vi "Komparator 4.0..vi"(10 "Q":u8, 11 "P":u8) -> (2 "P>Q":bool, 3 "P=Q":bool)   [LabVIEW 2020]
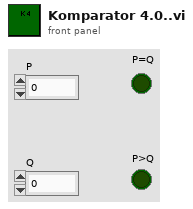
[diagram p1: front panel]
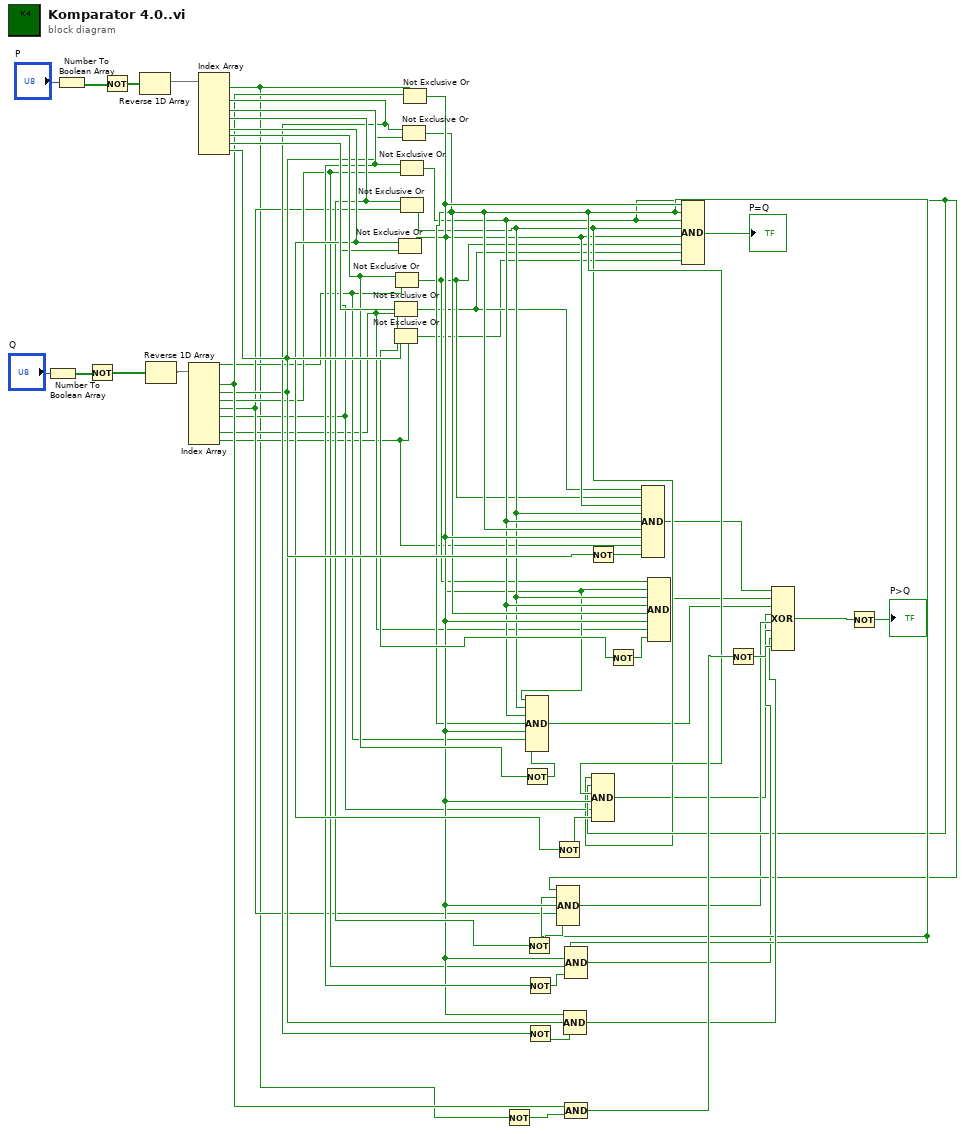
[diagram p0: block diagram]
diagram:
  n1 = Number To Boolean Array(number="Q") -> (Boolean array=w5:bool[])
  n2 = Number To Boolean Array(number="P") -> (Boolean array=w4:bool[])
  n3 = Not(x=w5) -> (.not. x?=w7:bool[])
  n4 = Not(x=w4) -> (.not. x?=w6:bool[])
  n5 = Reverse 1D Array(array=w6) -> (reversed array=w10:bool[])
  n6 = Reverse 1D Array(array=w7) -> (reversed array=w9:bool[])
  n7 = Index Array "Index Array"(array=w9) -> (element #1=w33:bool, element #2=w32:bool, element #3=w29:bool, element #4=w26:bool, element #5=w23:bool, element #6=w20:bool, element #7=w16:bool, element #8=w14:bool)  [unwired: 8 in]
  n8 = Index Array "Index Array"(array=w10) -> (element #1=w1:bool, element #2=w35:bool, element #3=w37:bool, element #4=w39:bool, element #5=w41:bool, element #6=w43:bool, element #7=w47:bool, element #8=w49:bool)  [unwired: 8 in]
  n9 = Not Exclusive Or(1:w16, 2:w47) -> (0:w13:bool)
  n10 = Not Exclusive Or(1:w14, 2:w49) -> (0:w11:bool)
  n11 = Not Exclusive Or(1:w20, 2:w43) -> (0:w15:bool)
  n12 = Not Exclusive Or(1:w23, 2:w41) -> (0:w19:bool)
  n13 = Not Exclusive Or(1:w29, 2:w37) -> (0:w25:bool)
  n14 = Not Exclusive Or(1:w26, 2:w39) -> (0:w22:bool)
  n15 = Not Exclusive Or(1:w32, 2:w35) -> (0:w28:bool)
  n16 = Not Exclusive Or(1:w33, 2:w1) -> (0:w31:bool)
  n17 = Not(x=w1) -> (.not. x?=w34:bool)
  n18 = Not(x=w43) -> (.not. x?=w44:bool)
  n19 = Not(x=w39) -> (.not. x?=w40:bool)
  n20 = Not(x=w37) -> (.not. x?=w38:bool)
  n21 = Not(x=w35) -> (.not. x?=w36:bool)
  n22 = Compound Arithmetic op=AND(w19, w22, w25, w28, w31, w20, w44) -> (w18:bool)
  n23 = Not(x=w41) -> (.not. x?=w42:bool)
  n24 = Compound Arithmetic op=AND(w25, w28, w31, w26, w40) -> (w24:bool)
  n25 = Compound Arithmetic op=AND(w31, w32, w36) -> (w30:bool)
  n26 = Compound Arithmetic op=AND(w28, w31, w29, w38) -> (w27:bool)
  n27 = Compound Arithmetic op=AND(w33, w34) -> (w45:bool)
  n28 = Not(x=w49) -> (.not. x?=w50:bool)
  n29 = Compound Arithmetic op=AND(w22, w25, w28, w31, w23, w42) -> (w21:bool)
  n30 = Not(x=w47) -> (.not. x?=w48:bool)
  n31 = Compound Arithmetic op=AND(w13, w15, w19, w22, w25, w28, w31, w14, w50) -> (w12:bool)
  n32 = Compound Arithmetic op=AND(w15, w19, w22, w25, w28, w31, w16, w48) -> (w17:bool)
  n33 = Compound Arithmetic op=AND(w31, w28, w25, w22, w19, w15, w13, w11) -> (→"P=Q":bool)
  n34 = Not(x=w45) -> (.not. x?=w46:bool)
  n35 = Compound Arithmetic op=XOR(w12, w17, w18, w21, w24, w27, w30, w46) -> (w51:bool)
  n36 = Not(x=w51) -> (.not. x?=→"P>Q":bool)
